vi "Math-Coerce Log Scale.vi"(0 "Value":dbl, 5 "Min":dbl, 7 "Max":dbl, 9 "Step":dbl) -> (4 "New Value":dbl)   [LabVIEW 2020]
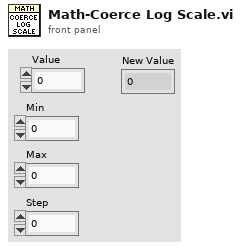
[diagram p1: front panel]
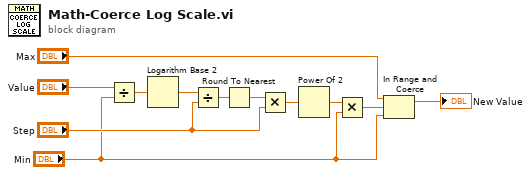
[diagram p0: block diagram]
diagram:
  n1 = Divide(x="Value", y="Min") -> (x/y=w9:dbl)
  n2 = Logarithm Base 2(1:w9) -> (0:w8:dbl)
  n3 = Divide(x=w8, y="Step") -> (x/y=w7:dbl)
  n4 = Round To Nearest(number=w7) -> (nearest integer value=w6:dbl)
  n5 = Multiply(x=w6, y="Step") -> (x*y=w4:dbl)
  n6 = Power Of 2(x=w4) -> (2^x=w3:dbl)
  n7 = Multiply(x=w3, y="Min") -> (x*y=w2:dbl)
  n8 = In Range and Coerce(upper limit="Max", x=w2, lower limit="Min") -> (coerced(x)=→"New Value":dbl)  [unwired: 1 out]
